vi "JAPCtiming3.vi"(8 "error in (no error)":errorcluster) -> (0 "error out":errorcluster)   [LabVIEW 2014]
uses:
  <userlib>/_RADE/RIO/JAPC/classes/JGet/openJAPCGet.vi
  <userlib>/_RADE/RIO/JAPC/classes/JGet/JAPCGet.vi
  <userlib>/_RADE/RIO/JAPC/classes/JGet/JGet.lvclass
panel:
  out "string":string
  out "double precision float":dbl format="%#_11g"
  in  "stop":bool
  out "data 2":dbl
  out "Instantaneous data":variant
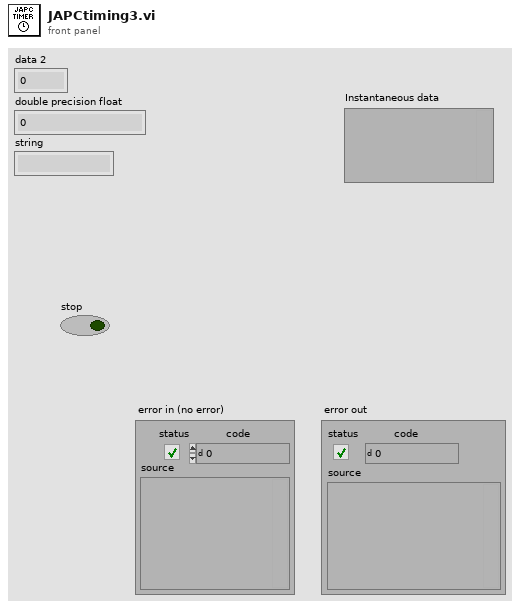
[diagram p1: front panel]
types:
  T1 = enum16{"open", "replace", "create", "open or create", "replace or create", "replace or create with confirmation"}
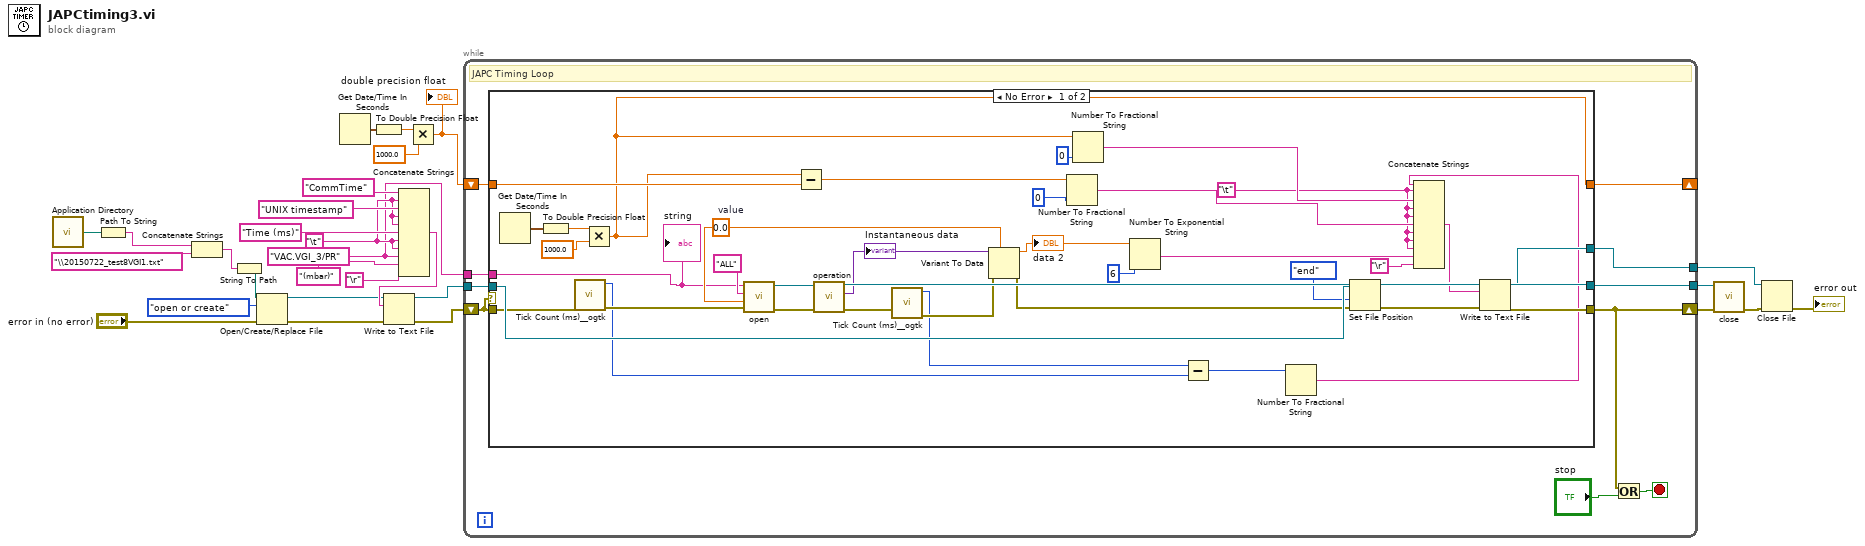
[diagram p0: block diagram]
diagram:
  w3 = "VAC.VGI_3/PR" ("string")
  w8 = "\t"
  n1 = call <vilib>:"Application Directory.vi"() -> ("Application Directory"=w21:path)
  n2 = Path To String(path=w21) -> (string=w20:string)
  n3 = Concatenate Strings(w20, "\\20150722_test8VGI1.txt" ("string")) -> (w17:string)
  n4 = String To Path(string=w17) -> (path=w18:path)
  n5 = Open/Create/Replace File(file path (use dialog)=w18, error in="error in (no error)", operation (0:open)=T1."open or create") -> (refnum out=w11:refnum<file>, error out=w12:errorcluster)  [unwired: 3 in, 1 out]
  n6 = Get Date/Time In Seconds() -> (seconds since 1Jan1904=w28:timestamp)
  n7 = To Double Precision Float(number=w28) -> (double precision float=w6:dbl)
  n8 = Concatenate Strings("CommTime" ("string"), w8, "UNIX timestamp" ("string"), w8, w8, "Time (ms)" ("string"), w8, w8, w3, "(mbar)" ("string"), "\r") -> (w15:string)
  n9 = Write to Text File(file (use dialog)=w11, text=w15, error in=w12) -> (refnum out=w10:refnum<file>, error out=w7:errorcluster)  [unwired: 1 in, 1 out]
  n10 = Multiply(x=w6, y=1000.0) -> (x*y=w4:dbl)
  "double precision float" <- w4
  n11 = while {
    tunnel: [w38] -> w27
    shift-right: [w36] -> w26
    shift-left: w7 -> [w35]
    tunnel: [w34] -> w16
    tunnel: w10 -> [w32]
    shift-right: [w31] -> _
    shift-left: w4 -> [w30]
    tunnel: w3 -> [w29]
    stop <- w37 stop-if-true
    # "JAPC Timing Loop"
    n12 = case shown="No Error" w35 {
      tunnel: [w76 _] -> w38
      tunnel: [w70 w79] -> w36
      tunnel: w35 -> [w44 w79]
      tunnel: w32 -> [w68 w78]
      tunnel: [w69 w78] -> w34
      tunnel: [w40 w77] -> w31
      tunnel: w30 -> [w54 w77]
      tunnel: w29 -> [w39 _]
      frame No Error {
        w51 = "\t"
        w75 = 0.0  # value
        n13 = Get Date/Time In Seconds() -> (seconds since 1Jan1904=w43:timestamp)
        n14 = To Double Precision Float(number=w43) -> (double precision float=w42:dbl)
        n15 = call <userlib>:"Tick Count (ms)__ogtk.vi"("error in (no error)"=w44) -> ("error out"=w50:errorcluster, "millisecond timer value"=w46:u32)  [unwired: 9 in]
        n16 = Multiply(x=w42, y=1000.0) -> (x*y=w40:dbl)
        n17 = call-poly <userlib>:"open.vi"("error in (no error)"=w50, "Data type"=w75, "Cycle"="ALL", "URL"=w39) -> ("error out"=w74:errorcluster, "Object out"=w73:refnum<class "JGet.lvclass">)  [unwired: 6 in]
        n18 = Subtract(x=w40, y=w54) -> (x-y=w53:dbl)
        n19 = call-poly <userlib>:"operation.vi"("error in (no error)"=w74, "Object in"=w73) -> ("error out"=w49:errorcluster, "Data"=w71:variant, "Object out"=w76:refnum<class "JGet.lvclass">)  [unwired: 5 in, 2 out]
        "Instantaneous data" <- w71
        n20 = call <userlib>:"Tick Count (ms)__ogtk.vi"("error in (no error)"=w49) -> ("error out"=w48:errorcluster, "millisecond timer value"=w47:u32)  [unwired: 9 in]
        n21 = Variant To Data(error in=w48, type=w75, Variant=w71) -> (data=w58:dbl, error out=w66:errorcluster)
        "data 2" <- w58
        n22 = Number To Fractional String(number=w53, precision (6)=i16 0) -> (F-format string=w52:string)  [unwired: 2 in]
        n23 = Number To Fractional String(number=w40, precision (6)=i16 0) -> (F-format string=w62:string)  [unwired: 2 in]
        n24 = Number To Exponential String(number=w58, precision (6)=i16 6) -> (E-format string=w45:string)  [unwired: 2 in]
        n25 = Subtract(x=w47, y=w46) -> (x-y=w60:u32)
        n26 = Number To Fractional String(number=w60) -> (F-format string=w59:string)  [unwired: 3 in]
        n27 = Set File Position(refnum=w68, from (0:start)=enum16{"start", "end", "current"}."end", error in=w66) -> (refnum out=w64:refnum<file>, error out=w65:errorcluster)  [unwired: 1 in]
        n28 = Concatenate Strings(w59, w51, w62, w51, w51, w52, w51, w51, w51, w45, "\r") -> (w61:string)
        n29 = Write to Text File(file (use dialog)=w64, text=w61, error in=w65) -> (refnum out=w69:refnum<file>, error out=w70:errorcluster)  [unwired: 1 in, 1 out]
        "string" <- w39
      }
      frame Error {
      }
    }
    n30 = Or(x=w36, y="stop") -> (x .or. y?=w37:bool)
  }
  n31 = call-dynamic "close.vi"("error in (no error)"=w26, "Object in"=w27) -> ("error out"=w25:errorcluster)  [unwired: 9 in]
  n32 = Close File(refnum=w16, error in=w25) -> (error out=→"error out":errorcluster)  [unwired: 1 out]
